vi "Broadcast Message.vi"(6 "timeout in ms (-1)":i32=-1, 8 "error in (no error)":errorcluster, 9 "Message in":refnum<class "Abstract Message.lvclass">, 11 "Abstract Producer in":refnum<class "Abstract Producer.lvclass">) -> (0 "error out":errorcluster, 1 "Messages out":refnum<class "Abstract Message.lvclass">[](array[class]), 3 "Abstract Producer out":refnum<class "Abstract Producer.lvclass">, 4 "timed out?":bool[](array[boolean]))   [LabVIEW 2027, in "Messaging.lvlib" / "Abstract Producer.lvclass"]
uses:
  Abstract Producer.lvclass
  Message/Abstract Message/Abstract Message.lvclass
  Abstract Producer.lvclass/Abstract Producer.ctl
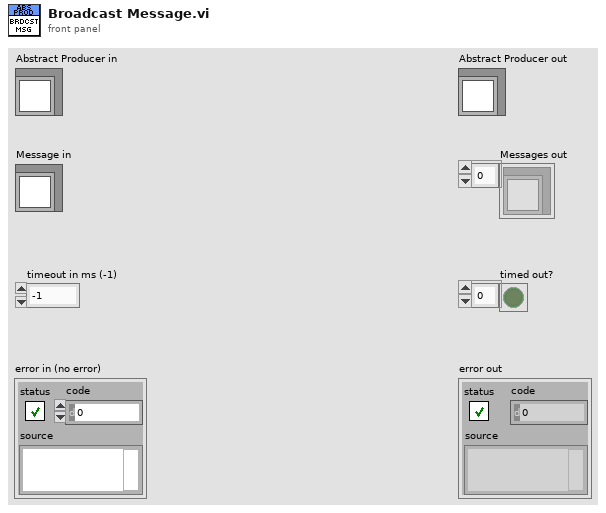
[diagram p1: front panel]
types:
  T1 = typedef "Messaging.lvlib/Abstract Producer.lvclass/Consumer Information.ctl" = cluster{"Name":string, "Request Queue":refnum<class "Abstract Message Queue.lvclass">, "Response Queue":refnum<class "Abstract Message Queue.lvclass">}
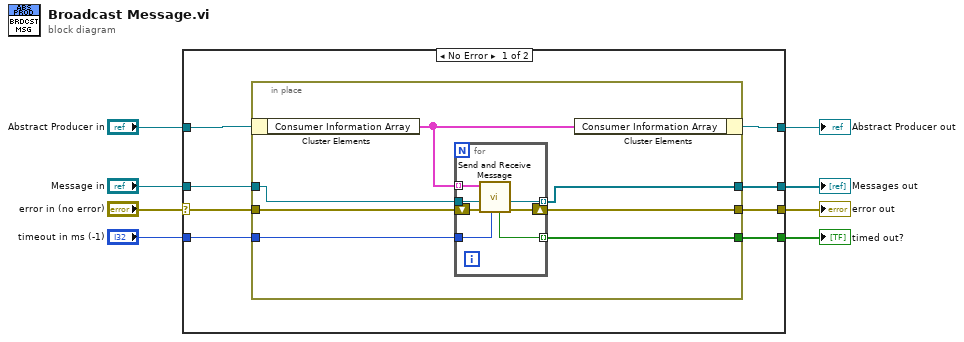
[diagram p0: block diagram]
diagram:
  n1 = case shown="No Error" "error in (no error)" {
    selector: "error in (no error)" -> [w16 w32]
    tunnel: [w15 w32] -> w7
    tunnel: [w12 w31] -> w5
    tunnel: "Abstract Producer in" -> [w14 w31]
    tunnel: "Message in" -> [w13 _]
    tunnel: "timeout in ms (-1)" -> [w10 _]
    tunnel: [w11 _] -> w2
    tunnel: [w9 _] -> w1
    frame No Error {
      n2 = in-place {
        in-place-border: w16 -> [w23]
        in-place-border: [w22] -> w15
        in-place-border: w13 -> [w20]
        in-place-border: [w19] -> w11
        in-place-border: w10 -> [w18]
        in-place-border: [w17] -> w9
        n3 = in-place-cluster #1(w14) -> ("Consumer Information Array"=w21:T1[])
        n4 = for {
          shift-right: [w29] -> w22
          shift-left: w23 -> [w30]
          tunnel: w21 -> [w28] mode=indexing
          tunnel: w20 -> [w27]
          tunnel: [w26] -> w17 mode=indexing
          tunnel: [w25] -> w19 mode=indexing
          tunnel: w18 -> [w24]
          n5 = call "Send and Receive Message.vi"("timeout in ms (-1)"=w24, "error in"=w30, "Message in"=w27, "Consumer Information"=w28) -> ("error out"=w29:errorcluster, "Message out"=w26:refnum<class "Abstract Message.lvclass">, "timed out?"=w25:bool)  [unwired: 5 in]
        }
        n6 = in-place-cluster #1("Consumer Information Array"=w21) -> (w12:refnum<class "Abstract Producer.lvclass">)
      }
    }
    frame Error {
    }
  }
  "error out" <- w7
  "Abstract Producer out" <- w5
  "timed out?" <- w2
  "Messages out" <- w1
